vi "Intialise Frames.vi"(8 "error in (no error)":errorcluster, 11 "ExperimentPath":path=path "C:/Users/All Other Users/Desktop/theo_videos/150610_15_33_59") -> (0 "error out":errorcluster, 1 "Experiment Parameters":T2, 2 "ROI setup":T1[](array[typedef]) {"Apparent Frame Size" format="%#_6f"; "Original FOV (um)" format="%#_6f"; "Pixels per miniscan" format="%#_6f"; "Dwell Time per pixel" format="%#_6f"; "Resolution" format="%#_6f"; "ROI group ID" format="%#_6f"; "Laser Power (%)" format="%#_6f"; "Zoom" format="%#_6f"; "Frame Size" format="%#_6f"; "Number of lines" format="%#_6f"; "Composite ID" format="%#_6f"; "Angle (deg)" format="%#_6f"; "ROI Time (ns)" format="%#_6f"; "ROI ID" format="%#_6f"; "Pixels in ROI" format="%#_6f"; "ROI index" format="%#_6f"; "Z stop" format="%#_6f"; "Y stop" format="%#_6f"; "X stop" format="%#_6f"; "Z start" format="%#_6f"; "X start" format="%#_6f"; "Y start" format="%#_6f"}, 3 "TDMS references(All Trials)":refnum<k34>[](array[refnum]))   [LabVIEW 2020]
uses:
  Typedefs/Experiment Parameters.ctl
  Functional Imaging Viewer/Typedefs/ROI parameters data type.ctl
  Functional Imaging Viewer/SubVIs/Experiment header interface/Typedefs/Header file interface module functions enum.ctl
  Functional Imaging Viewer/SubVIs/Experiment header interface/Typedefs/Header file type enum.ctl
panel:
  out "All Trials TDMS Exists":bool
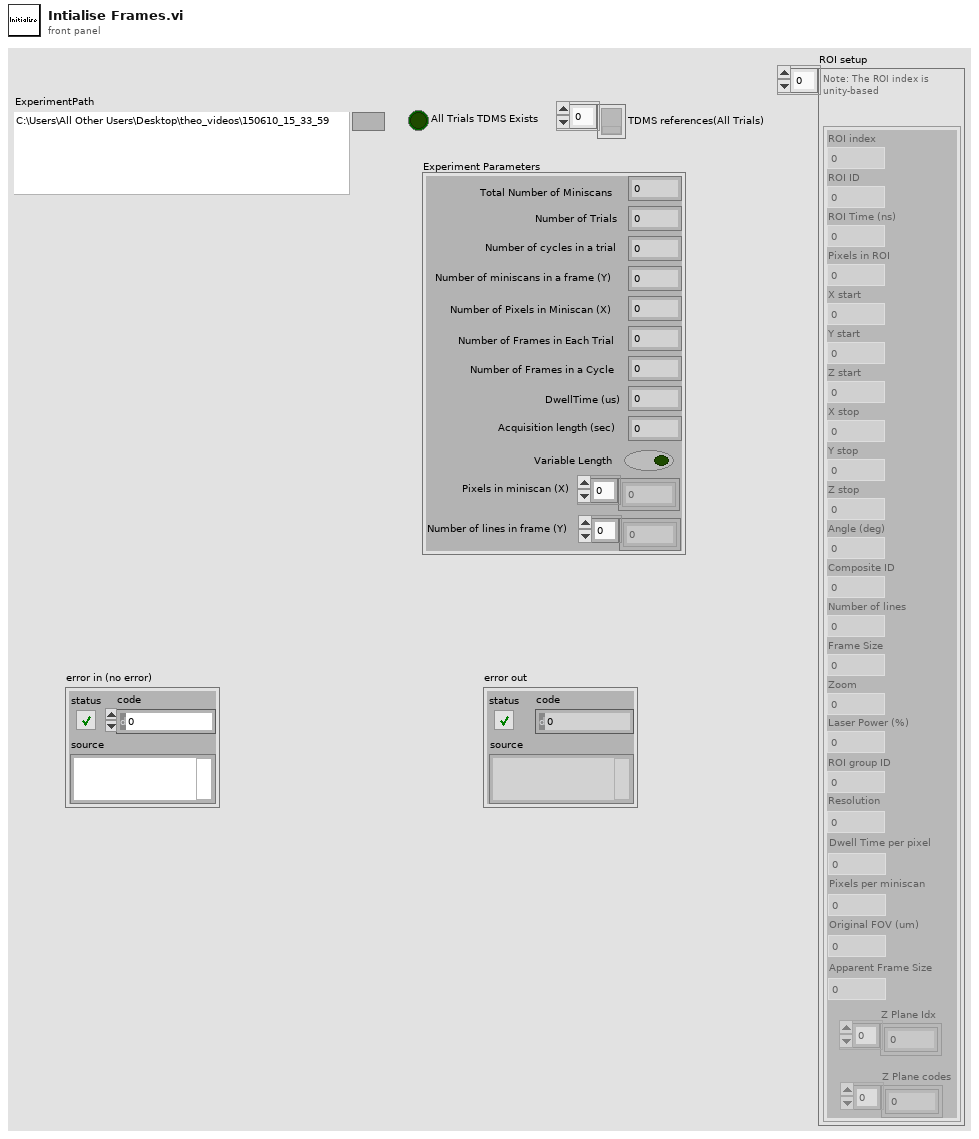
[diagram p1: front panel]
types:
  T1 = typedef "ROI parameters data type.ctl" = cluster{"ROI index":dbl, "ROI ID":dbl, "ROI Time (ns)":dbl, "Pixels in ROI":dbl, "X start":dbl, "Y start":dbl, "Z start":dbl, "X stop":dbl, "Y stop":dbl, "Z stop":dbl, "Angle (deg)":dbl, "Composite ID":dbl, "Number of lines":dbl, "Frame Size":dbl, "Zoom":dbl, "Laser Power (%)":dbl, "ROI group ID":dbl, "Resolution":dbl, "Dwell Time per pixel":dbl, "Pixels per miniscan":dbl, "Original FOV (um)":dbl, "Apparent Frame Size":dbl, "Z Plane Idx":i32[], "Z Plane codes":i32[]}
  T2 = typedef "Experiment Parameters.ctl" = cluster{"Total Number of Miniscans":i32, "Number of Trials":i32, "Number of cycles in a trial":i32, "Number of miniscans in a frame (Y)":i32, "Number of Pixels in Miniscan (X)":i32, "Number of Frames in Each Trial":i32, "Number of Frames in a Cycle":i32, "DwellTime (us)":dbl, "Acquisition length (sec)":dbl, "Variable Length":bool, "Pixels in miniscan (X)":dbl[], "Number of lines in frame (Y)":dbl[]}
  T3 = typedef "Header file interface module functions enum.ctl" = enum16{"Load experiment header file", "Save experiment header file", "Clear stored values", "Read stored values", "Update specific value in memory", "Update values in memory"}
  T4 = typedef "Header file type enum.ctl" = enum16{"All parameters", "Params for funct acq w ROI or mscn", "Params for funct acq w rectangles", "Live imaging header parameters", "AOL Parameters"}
  T5 = typedef "Header parameters cluster-ALL.ctl" = cluster{"LOGIN":T6, "GLOBAL PARAMETERS":T7, "IMAGING MODES":T9, "TIME SERIES":T10, "MOTOR Z-STACK ":T13, "AOL Z-STACK":T14, "FUNCTIONAL IMAGING":T15, "VOLUME IMAGING":T15, "MOVEMENT CORRECTION":T19, "CALIBRATION":T21, "STATISTICS":T22, "BIOLOGY INFORMATION":T23, "Calibration Data":T24}
  T6 = typedef "Header params -Login.ctl" = cluster{"User":string, "Profile":string, "Software Version":string, "Experiment Date Time":timestamp}
  T7 = typedef "Header params-Global Parameters.ctl" = cluster{"MicroscopeID":string, "Microscope Type":string, "Objective":string, "Field of View (um)":dbl, "Fill time (us)":dbl, "Experiment Type":T8, "Stimuli Trigger":bool, "Speed Logging":bool}
  T8 = typedef "Experiment Type.ctl" = enum16{"In vivo", "In vitro", "Testing", "Calibration", "Other"}
  T9 = typedef "Header params-Imaging Modes.ctl" = cluster{"Time Series":bool, "Motor Zstack":bool, "AOL Zstack":bool, "Functional Imaging":bool, "Volume Imaging":bool}
  T10 = typedef "Header params-Time Series.ctl" = cluster{"Basic Image meta data":T11, "AOL z":dbl}
  T11 = typedef "Header params-Basic image meta data.ctl" = cluster{"Wavelength (nm)":dbl, "# averaged frames":dbl, "laser power (%)":dbl, "Pockels":dbl, "pixel dwell time (us)":dbl, "pmt 1":dbl, "pmt 2":dbl, "back apperture":dbl, "zoom":dbl, "field of view":dbl, "Frame Size":T12, "AOL x centre":dbl, "AOL y centre":dbl, "Stage x position":dbl, "Stage y position":dbl, "Stage z position":dbl}
  T12 = typedef "Frame Size.ctl" = u16
  T13 = typedef "Header params-Motor Z-stack.ctl" = cluster{"Hdr Basic Image meta data":T11, "Z Start":dbl, "Z Stop":dbl, "No of Planes":i32, "Laser Power (%) at Z Start":dbl, "Laser Power (%) at Z Stop":dbl}
  T14 = typedef "Header params-AOL Z-stack.ctl" = cluster{"Hdr Basic Image meta data":T11, "Z Start":dbl, "Z Stop":dbl, "No of Planes":i32, "Laser Power (%) at Z Start":dbl, "Laser Power (%) at Z Stop":dbl}
  T15 = typedef "Header params-Functional Imaging.ctl" = cluster{"Functional Mode":T16, "Variable Length":bool, "Variable Resolution":bool, "Pockels Modulation":bool, "Stimuli Trigger":bool, "Cool down enabled":bool, "AOL Mode":T17, "Plane Mode":T18, "Miniscan Dwell time per pixel (us)":dbl, "poi dwell time":dbl, "Number of trials":dbl, "Number of cycles":dbl, "Number of pois":dbl, "Number of miniscans":dbl, "Number of pixels in miniscan":dbl, "Rectangle ROI length":dbl, "Rectangle ROI height":dbl, "Frame rate (fps)":dbl, "Acquisition Length":dbl, "video length (sec)":dbl, "Stimuli delay (sec)":dbl, "Cool down time (sec)":dbl, "Basic Image meta data":T11, "Z Start (um)":dbl, "Z Stop (um)":dbl}
  T16 = typedef "Functional Mode.ctl" = enum16{"Point", "Line", "Patch", "Plane", "Volume"}
  T17 = typedef "AOL modes.ctl" = enum16{"Raster", "Structural", "Pointing", "Mini Scan", "Alignment"}
  T18 = typedef "Plane Mode.ctl" = u16
  T19 = typedef "Header params-Movement correction.ctl" = cluster{"Movement Correction":bool, "Axial Reference":bool, "Reference Source":T20, "Full Frame Size":dbl, "Reference Field of View":dbl, "Reference Zoom":dbl, "Reference dwell time (us)":dbl, "Reference X Pixels":dbl, "Reference Y Pixels":dbl, "Number of Z lines":dbl, "Size of Z pixels":dbl, "Axial Pixels":dbl, "Ignore Z lines":dbl, "Reference Scan Cycles":dbl, "Reference Threshold XY":dbl, "Reference Threshold Z":dbl, "Reference Average XY":dbl, "Reference Average Z":dbl, "Proportional Scale":dbl, "Integral Scale":dbl, "Proportional Scale Z":dbl, "Integral Scale Z":dbl, "Diff Threshold":dbl, "Diff Threshold Z":dbl, "Sliding Average":bool, "Reference count reset enabled":bool, "Scan Interval (ms)":dbl, "Ref Plot Refresh Rate (ms)":dbl}
  T20 = typedef "Reference source.ctl" = enum16{"Green channel", "Red channel"}
  T21 = typedef "Header params-Calibration Setup.ctl" = cluster{"Pockels Calibration File":path, "Calibration_ini file":path, "Setup_ini file":path}
  T22 = typedef "Header params-statistics.ctl" = cluster{"Z-stack duration (sec)":dbl, "Number of acquired data-points":dbl, "Acquisition time (ms)":dbl, "Number of acquired frames":dbl, "Intertrial times":dbl[]}
  T23 = typedef "Biology Information.ctl" = cluster{"Animal Code or Name":string, "Animal DoB":string, "Animal Age":string, "Animal Sex":string, "Animal Weight":string, "Date of Injection":string, "Date of Implant":string, "Site of Injection":string, "Animal Ear Notch":string, "AAV constructs":string, "Genetic background":string, "Optical reporter":string, "Region of brain imaged":string, "Other \ncomments":string}
  T24 = typedef "Header params-calibration data.ctl" = cluster{"Objective Name":string, "Calibration Wavelength":dbl, "Sum X":dbl, "Sum Y":dbl, "Diff X":dbl, "Diff Y":dbl, "Distortion Correction":dbl, " Z norm to um Scaling":dbl, " X norm to um Scaling":dbl}
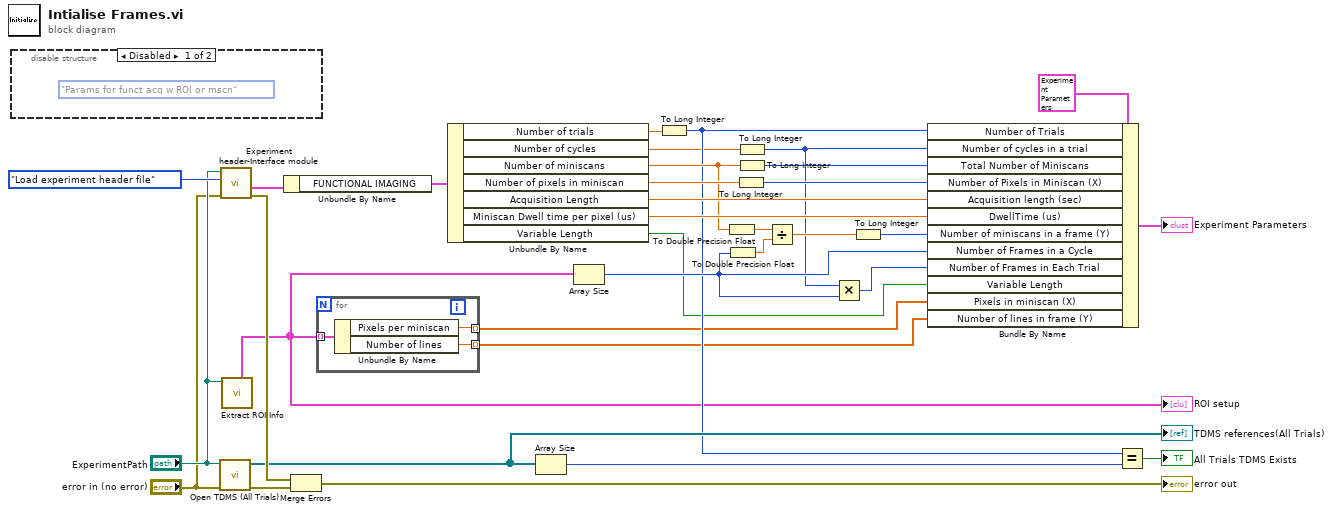
[diagram p0: block diagram]
diagram:
  n1 = disable-structure shown="Disabled" {
    frame Disabled {
      (unwired) Header_file_type_enum."Params for funct acq w ROI or mscn" ("Header file type")
    }
    frame Enabled {
    }
  }
  n2 = call "Open TDMS (All Trials).vi"("error in (no error)"="error in (no error)", "Experiment Folder"="ExperimentPath") -> ("error out"=w25:errorcluster, "TDMS references(All Trials)"=w18:refnum<k34>[])  [unwired: 7 in, 1 out]
  "TDMS references(All Trials)" <- w18
  n3 = call "Experiment header-Interface module.vi"("error in (no error)"="error in (no error)", "Function"=Header_file_interface_module_functions_enum."Load experiment header file", "Experiment data folder path"="ExperimentPath") -> ("error out"=w26:errorcluster, "All header parameters out"=w10:T5)  [unwired: 7 in]
  n4 = call "Extract ROI Info.vi"("AVI File Path"="ExperimentPath") -> ("ROI setup"=w4:T1[])  [unwired: 7 in, 3 out]
  "ROI setup" <- w4
  n5 = Unbundle By Name(w10) -> ("FUNCTIONAL IMAGING"=w9:T15)
  n6 = Merge Errors(w26, w25) -> (→"error out":errorcluster)
  n7 = for {
    tunnel: w4 -> [w36] mode=indexing
    tunnel: [w35] -> w3 mode=indexing
    tunnel: [w34] -> w2 mode=indexing
    n8 = Unbundle By Name(w36) -> ("Pixels per miniscan"=w35:dbl, "Number of lines"=w34:dbl)
  }
  n9 = Unbundle By Name(w9) -> ("Number of trials"=w8:dbl, "Number of cycles"=w5:dbl, "Number of miniscans"=w17:dbl, "Number of pixels in miniscan"=w19:dbl, "Acquisition Length"=w22:dbl, "Miniscan Dwell time per pixel (us)"=w21:dbl, "Variable Length"=w1:bool)
  n10 = Array Size(array=w18) -> (size(s)=w29:i32)
  n11 = Array Size(array=w4) -> (size(s)=w15:i32)
  n12 = To Long Integer(number=w8) -> (32bit integer=w7:i32)
  n13 = To Double Precision Float(number=w17) -> (double precision float=w31:dbl)
  n14 = To Double Precision Float(number=w15) -> (double precision float=w30:dbl)
  n15 = To Long Integer(number=w19) -> (32bit integer=w14:i32)
  n16 = To Long Integer(number=w5) -> (32bit integer=w6:i32)
  n17 = To Long Integer(number=w17) -> (32bit integer=w12:i32)
  n18 = Divide(x=w31, y=w30) -> (x/y=w20:dbl)
  n19 = Multiply(x=w6, y=w15) -> (x*y=w16:i32)
  n20 = To Long Integer(number=w20) -> (32bit integer=w13:i32)
  n21 = Bundle By Name(cluster=T2 {"Total Number of Miniscans"=10, "Number of Trials"=260, "Number of cycles in a trial"=1005, "Number of miniscans in a frame (Y)"=138, "Number of Pixels in Miniscan (X)"=10, "Number of Frames in Each Trial"=0, "Number of Frames in a Cycle"=67, "DwellTime (us)"=0.0, "Acquisition length (sec)"=0.0, "Variable Length"=FALSE, "Pixels in miniscan (X)"=[], "Number of lines in frame (Y)"=[]} ("Experiment Parameters"), "Number of Trials"=w7, "Number of cycles in a trial"=w6, "Total Number of Miniscans"=w12, "Number of Pixels in Miniscan (X)"=w14, "Acquisition length (sec)"=w22, "DwellTime (us)"=w21, "Number of miniscans in a frame (Y)"=w13, "Number of Frames in a Cycle"=w15, "Number of Frames in Each Trial"=w16, "Variable Length"=w1, "Pixels in miniscan (X)"=w3, "Number of lines in frame (Y)"=w2) -> (→"Experiment Parameters":T2)
  n22 = Equal?(x=w7, y=w29) -> (x = y?=→"All Trials TDMS Exists":bool)
